vi "Unregister and Close Sessions.vi"(8 "error in":errorcluster) -> (0 "error out":errorcluster)   [LabVIEW 2024, in "NIFgenSignalVoltageGeneration.lvlib"]
uses:
  NIFgenSignalVoltageGeneration.lvlib
  <vilib>/MeasurementLink/MeasurementLink niFGEN/MeasurementLink niFGEN.lvlib
  <vilib>/MeasurementLink/MeasurementLink niFGEN/Initialize Sessions - NSess.vi
  <vilib>/MeasurementLink/MeasurementLink Session Management V1/Session Reservation/Session Reservation.lvclass
  <vilib>/MeasurementLink/MeasurementLink Session Management V1/Session Reservation/Initialize and Close Session Behavior.ctl
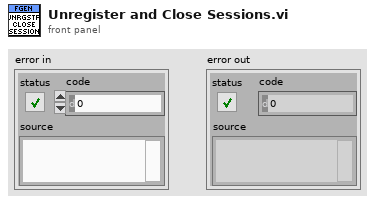
[diagram p1: front panel]
types:
  T1 = typedef "MeasurementLink Session Management V1.lvlib/Session Reservation.lvclass/Initialize and Close Session Behavior.ctl" = enum16{"Auto", "Initialize and Close", "Attach and Detach", "Initialize and Detach", "Attach and Close"}
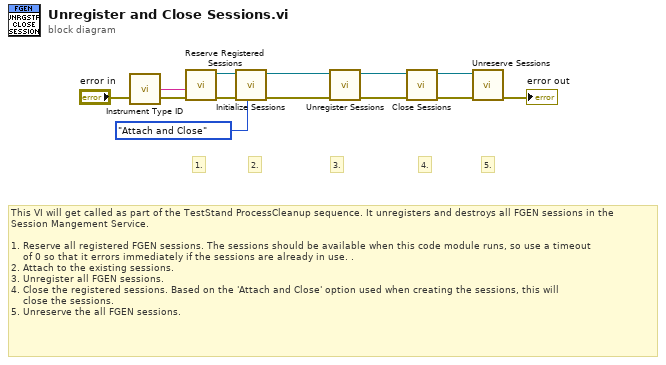
[diagram p0: block diagram]
diagram:
  # "5."
  # "4."
  # "3."
  # "2."
  # "1."
  # "This VI will get called as part of the TestStand ProcessCleanup sequence. It unregisters and destroys all FGEN sessions in the\nSession Mangement Service.\n\n1. Reserve all registered FGEN sessions. The sessions should be available when this code module runs, so use a timeout\n    of 0 so that it errors immediately if the sessions are already in use. .\n2. Attach to the existing sessions.\n3. Unregister all FGEN sessions.\n4. Close the registered sessions. Based on the 'Attach and Close' option used when creating the sessions, this will\n    close the sessions.\n5. Unreserve the all FGEN sessions."
  n1 = call <vilib>:"Instrument Type ID.vi"() -> ("instrument type id"=w7:string)  [unwired: 5 in]
  n2 = call <vilib>:"Reserve Registered Sessions.vi"("error in"="error in", "instrument type id"=w7) -> ("error out"=w12:errorcluster, "session reservation out"=w11:refnum<class "Session Reservation.lvclass">)  [unwired: 8 in]
  n3 = call-poly <vilib>:"Initialize Sessions.vi"("initialize and close session behavior"=Initialize_and_Close_Session_Behavior."Attach and Close", "error in"=w12, "session reservation in"=w11) -> ("error out"=w6:errorcluster, "session reservation out"=w10:refnum<class "Session Reservation.lvclass">)  [unwired: 5 in, 2 out]
  n4 = call <vilib>:"Unregister Sessions.vi"("error in"=w6, "session reservation in"=w10) -> ("error out"=w2:errorcluster, "session reservation out"=w4:refnum<class "Session Reservation.lvclass">)  [unwired: 8 in]
  n5 = call <vilib>:"Close Sessions.vi"("error in"=w2, "session reservation in"=w4) -> ("error out"=w1:errorcluster, "session reservation out"=w3:refnum<class "Session Reservation.lvclass">)  [unwired: 8 in]
  n6 = call <vilib>:"Unreserve Sessions.vi"("error in"=w1, "session reservation in"=w3) -> ("error out"=→"error out":errorcluster)  [unwired: 9 in]
